vi "Read.vi"(5 "Username":string, 6 "Password":string, 7 "Address":string, 8 "Error In":errorcluster) -> (0 "Error Out":errorcluster)   [LabVIEW 2018, in "Tests.lvlib" / "SFTP Directory.lvlib"]
uses:
  SFTP Directory.lvlib
  src/Toolkit/API/SFTP File/API/Typedefs/Flags.ctl
  src/Toolkit/API/SFTP Attributes/Support/Create from SFTP Directory.vi
  src/Toolkit/API/SFTP Attributes/Support/Destroy to SFTP Directory.vi
  <vilib>/addons/_JKI Toolkits/Caraya/classes/Test/Test.lvclass
  <vilib>/addons/_JKI Toolkits/Caraya/classes/Assert/Assert.lvclass
  src/Toolkit/API/SFTP Directory/SFTP Directory.lvclass
  src/Toolkit/API/SFTP Attributes/SFTP Attributes.lvclass
  src/Toolkit/API/SFTP File/SFTP File.lvclass
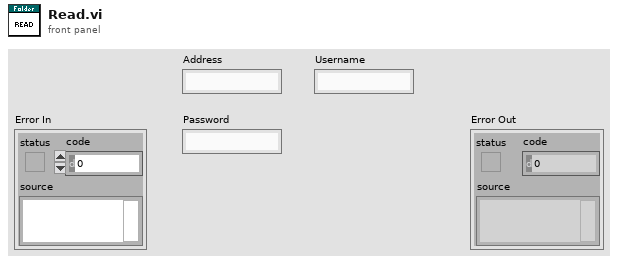
[diagram p1: front panel]
types:
  T1 = typedef "Toolkit.lvlib/SFTP File.lvclass/Flags.ctl" = cluster{"Read":bool, "Write":bool, "Append":bool, "Create":bool, "Truncate":bool, "Exclude":bool}
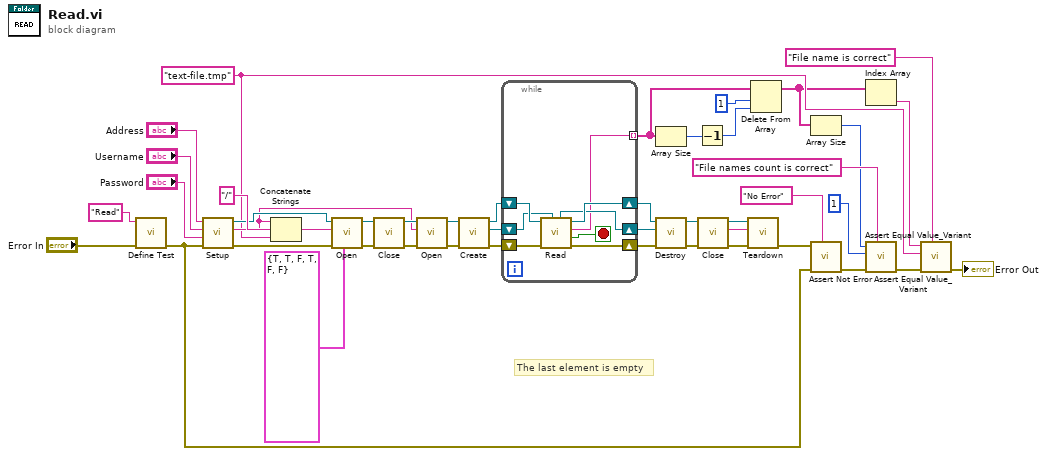
[diagram p0: block diagram]
diagram:
  w6 = "text-file.tmp"
  # "The last element is empty"
  n1 = call <vilib>:"Define Test.vi"("error in (no error)"="Error In", "Label (VI Title)"="Read") -> ("error out"=w36:errorcluster)  [unwired: 9 in]
  n2 = call "Setup.vi"("Error In"=w36, "Password"="Password", "Username"="Username", "Address"="Address") -> ("Error Out"=w23:errorcluster, "Temporary Directory"=w17:string, "SFTP"=w22:refnum<class "SFTP.lvclass">)  [unwired: 5 in]
  n3 = Concatenate Strings(w17, "/", w6) -> (w25:string)
  n4 = call "Open.vi"("Flags"=T1 {"Read"=TRUE, "Write"=TRUE, "Append"=FALSE, "Create"=TRUE, "Truncate"=FALSE, "Exclude"=FALSE}, "Error In"=w23, "Remote Path"=w25, "SFTP"=w22) -> ("Error Out"=w20:errorcluster, "SFTP File"=w21:refnum<class "SFTP File.lvclass">)  [unwired: 6 in]
  n5 = call "Close.vi"("Error In"=w20, "SFTP File"=w21) -> ("Error Out"=w18:errorcluster, "SFTP"=w19:refnum<class "SFTP.lvclass">)  [unwired: 7 in, 1 out]
  n6 = call "Open.vi"("Error In"=w18, "Remote Path"=w17, "SFTP"=w19) -> ("Error Out"=w11:errorcluster, "SFTP Directory"=w15:refnum<class "SFTP Directory.lvclass">)  [unwired: 7 in]
  n7 = call-poly "Create.vi"("Error In"=w11, "SFTP Directory In"=w15) -> ("Error Out"=w12:errorcluster, "SFTP Attributes"=w13:refnum<class "SFTP Attributes.lvclass">, "SFTP Directory Out"=w14:refnum<class "SFTP Directory.lvclass">)  [unwired: 7 in]
  n8 = while {
    shift-right: [w50] -> w31
    shift-left: w14 -> [w49]
    shift-right: [w52] -> w28
    shift-left: w12 -> [w51]
    shift-right: [w48] -> w29
    shift-left: w13 -> [w46]
    tunnel: [w47] -> w4 mode=indexing
    stop <- w53 stop-if-true
    n9 = call "Read.vi"("SFTP Attributes In"=w46, "Error In"=w51, "SFTP Directory In"=w49) -> ("Error Out"=w52:errorcluster, "End-of-File?"=w53:bool, "File Name"=w47:string, "SFTP Directory Out"=w50:refnum<class "SFTP Directory.lvclass">, "SFTP Attributes Out"=w48:refnum<class "SFTP Attributes.lvclass">)  [unwired: 4 in]
  }
  n10 = Array Size(array=w4) -> (size(s)=w3:i32)
  n11 = call-poly "Destroy.vi"("Error In"=w28, "SFTP Attributes"=w29, "SFTP Directory In"=w31) -> ("Error Out"=w27:errorcluster, "SFTP Directory Out"=w30:refnum<class "SFTP Directory.lvclass">)  [unwired: 7 in]
  n12 = Decrement(x=w3) -> (x-1=w2:i32)
  n13 = call "Close.vi"("Error In"=w27, "SFTP Directory"=w30) -> ("Error Out"=w34:errorcluster, "Remote Path"=w16:string, "SFTP"=w32:refnum<class "SFTP.lvclass">)  [unwired: 7 in]
  n14 = call "Teardown.vi"("Error In"=w34, "Temporary Directory"=w16, "SFTP"=w32) -> ("Error Out"=w35:errorcluster)  [unwired: 8 in]
  n15 = Delete From Array(array=w4, length=1, index=w2) -> (array with subset deleted=w1:string[])  [unwired: 1 out]
  n16 = Array Size(array=w1) -> (size(s)=w33:i32)
  n17 = call <vilib>:"Assert Not Error.vi"("Label"="No Error", "error in (no error)"=w36, "Not Error?"=w35) -> ("error out"=w42:errorcluster)  [unwired: 8 in]
  n18 = Index Array(array=w1) -> (element=w7:string)  [unwired: 1 in]
  n19 = call <vilib>:"Assert Equal Value_Variant.vi"("Label"="File names count is correct", "error in (no error)"=w42, "Y"=1 ("size(s)"), "X"=w33) -> ("error out"=w10:errorcluster)  [unwired: 7 in]
  n20 = call <vilib>:"Assert Equal Value_Variant.vi"("Label"="File name is correct", "error in (no error)"=w10, "Y"=w6, "X"=w7) -> ("error out"=→"Error Out":errorcluster)  [unwired: 7 in]
